vi "KE6221 -- Set Arm Layer Trig Layer Wave Trig Params.vi"(0 "Resource In":refnum<visa-resource-name>, 1 "Check For SCPI Errors? (T)":bool=TRUE, 7 "6221 Arm Trig Wave Trig Params In":T1={"Arm Layer Input Trig Bypassed?"=FALSE, "Arm Layer Input Trig Source"=enum."Immediate", "Arm Layer Input Trig Link Line"=enum."1", "Arm Layer Input Trig Timer Interval (s)"=0.001, "Arm Layer Output Trig Mode"=enum."No Trig Out", "Arm Layer Output Trig Link Line"=enum."1", "Trig Layer Input Trig Source"=enum."Immediate", "Trig Layer Input Trig Link Line"=enum."1", "Trig Layer Output Trig Mode"=enum."No Trig Out", "Trig Layer Output Trig Link Line"=enum."1", "6221 Wave Input Trig Enabled?"=FALSE, "6221 Wave Input Trig Link Line"=enum."None", "6221 Wave Inactive Level (%)"=0.0, "6221 Wave Ingore Input Retrigs?"=FALSE, "6221 Phase Marker Output Trig Enabled?"=FALSE, "6221 Phase Marker (deg)"=180.0, "6221 Phase Marker Output Trig Link Line"=enum."6"} {"6221 Phase Marker (deg)" min=0.0 max=360.0 format="%.3f"; "6221 Wave Inactive Level (%)" min=-100.0 max=100.0 format="%.3p"; "Arm Layer Input Trig Timer Interval (s)" min=0.001 max=99999.999 step=0.001 format="%.3f"}, 11 "error in (no error)":errorcluster) -> (4 "Resource Out (dupl)":refnum<visa-resource-name>, 8 "6221 Arm Trig Wave Trig Params Out":T1={"Arm Layer Input Trig Bypassed?"=FALSE, "Arm Layer Input Trig Source"=enum."Immediate", "Arm Layer Input Trig Link Line"=enum."1", "Arm Layer Input Trig Timer Interval (s)"=0.001, "Arm Layer Output Trig Mode"=enum."No Trig Out", "Arm Layer Output Trig Link Line"=enum."1", "Trig Layer Input Trig Source"=enum."Immediate", "Trig Layer Input Trig Link Line"=enum."1", "Trig Layer Output Trig Mode"=enum."No Trig Out", "Trig Layer Output Trig Link Line"=enum."1", "6221 Wave Input Trig Enabled?"=FALSE, "6221 Wave Input Trig Link Line"=enum."None", "6221 Wave Inactive Level (%)"=0.0, "6221 Wave Ingore Input Retrigs?"=FALSE, "6221 Phase Marker Output Trig Enabled?"=FALSE, "6221 Phase Marker (deg)"=180.0, "6221 Phase Marker Output Trig Link Line"=enum."6"} {"6221 Phase Marker (deg)" min=0.0 max=360.0 format="%.3f"; "6221 Wave Inactive Level (%)" min=-100.0 max=100.0 format="%.3p"; "Arm Layer Input Trig Timer Interval (s)" min=0.001 max=99999.999 step=0.001 format="%.3f"}, 15 "error out":errorcluster)   [LabVIEW 2018, in "Keithley 622x.lvlib"]
doc: "Sets the parameters for the 'Arm' and 'Trigger' layers of the trigger model, and also the trigger parameters for waveform playback. Note that this VI can only be used with the 6221, since the 6220 doesn't support waveform playback."
uses:
  Keithley 622x.lvlib
  Low Level/Typedefs/KE622x -- Trig Source.ctl
  Low Level/Typedefs/KE622x -- Trig Link Line.ctl
  Low Level/Typedefs/KE622x -- Trig Output Mode.ctl
  Low Level/Typedefs/KE622x -- Arm Source.ctl
  Low Level/Typedefs/KE622x -- Arm Output Mode.ctl
  Low Level/Typedefs/KE622x -- Arm Timer Interval.ctl
  6221 Wave/Low Level/Typedefs/KE6221 -- Wave Extern Trig Link In Line.ctl
  6221 Wave/Low Level/Typedefs/KE6221 -- Wave Inactive Level.ctl
  6221 Wave/Low Level/Typedefs/KE6221 -- Wave Phase Marker.ctl
  Typedefs/KE6221 -- Arm Trig Wave Trig Params.ctl
panel:
  out "Num Errors":u32
  out "Errors":string[](array[string])
  # "Arm Layer"
  # "Trig Layer"
  # "KE6221 Wave"
  # "Arm Layer"
  # "Trig Layer"
  # "KE6221 Wave"
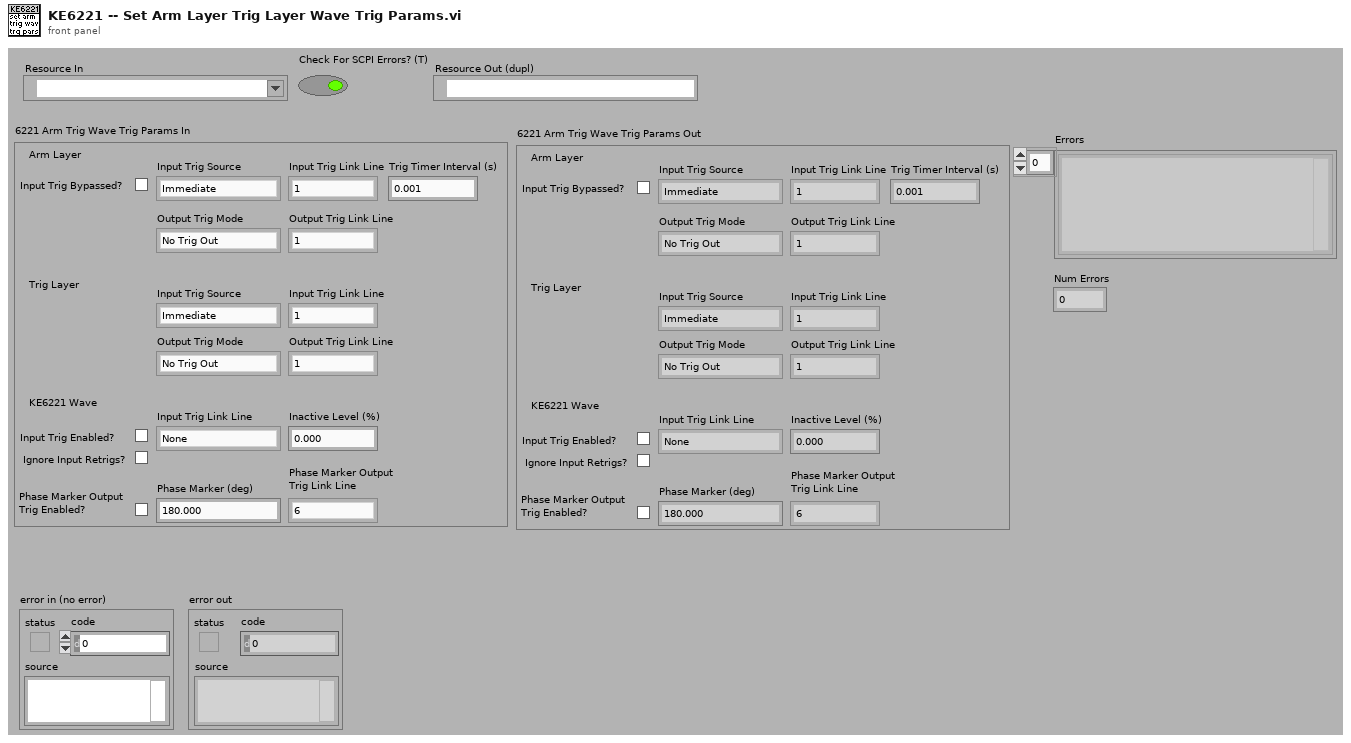
[diagram p1: front panel]
types:
  T1 = typedef "Keithley 622x.lvlib/KE6221 -- Arm Trig Wave Trig Params.ctl" = cluster{"Arm Layer Input Trig Bypassed?":bool, "Arm Layer Input Trig Source":T2, "Arm Layer Input Trig Link Line":T3, "Arm Layer Input Trig Timer Interval (s)":T4, "Arm Layer Output Trig Mode":T5, "Arm Layer Output Trig Link Line":T3, "Trig Layer Input Trig Source":T6, "Trig Layer Input Trig Link Line":T3, "Trig Layer Output Trig Mode":T7, "Trig Layer Output Trig Link Line":T3, "6221 Wave Input Trig Enabled?":bool, "6221 Wave Input Trig Link Line":T8, "6221 Wave Inactive Level (%)":T9, "6221 Wave Ingore Input Retrigs?":bool, "6221 Phase Marker Output Trig Enabled?":bool, "6221 Phase Marker (deg)":T10, "6221 Phase Marker Output Trig Link Line":T3}
  T2 = typedef "Keithley 622x.lvlib/KE622x -- Arm Source.ctl" = enum16{"Immediate", "Bus (*TRG)", "Timer", "Manual", "Trigger Link", "SOT Falling Edge", "SOT Rising Edge", "SOT Either Edge"}
  T3 = typedef "Keithley 622x.lvlib/KE622x -- Trig Link Line.ctl" = enum16{"1", "2", "3", "4", "5", "6"}
  T4 = typedef "Keithley 622x.lvlib/KE622x -- Arm Timer Interval.ctl" = dbl
  T5 = typedef "Keithley 622x.lvlib/KE622x -- Arm Output Mode.ctl" = enum16{"No Trig Out", "Trig Out On Enter Arm", "Trig Out On Exit Arm"}
  T6 = typedef "Keithley 622x.lvlib/KE622x -- Trig Source.ctl" = enum16{"Immediate", "Trigger Link"}
  T7 = typedef "Keithley 622x.lvlib/KE622x -- Trig Output Mode.ctl" = enum16{"No Trig Out", "Source Turn On", "After Source Delay"}
  T8 = typedef "Keithley 622x.lvlib/KE6221 -- Wave Extern Trig Link In Line.ctl" = enum16{"None", "1", "2", "3", "4", "5", "6"}
  T9 = typedef "Keithley 622x.lvlib/KE6221 -- Wave Inactive Level.ctl" = dbl
  T10 = typedef "Keithley 622x.lvlib/KE6221 -- Wave Phase Marker.ctl" = dbl
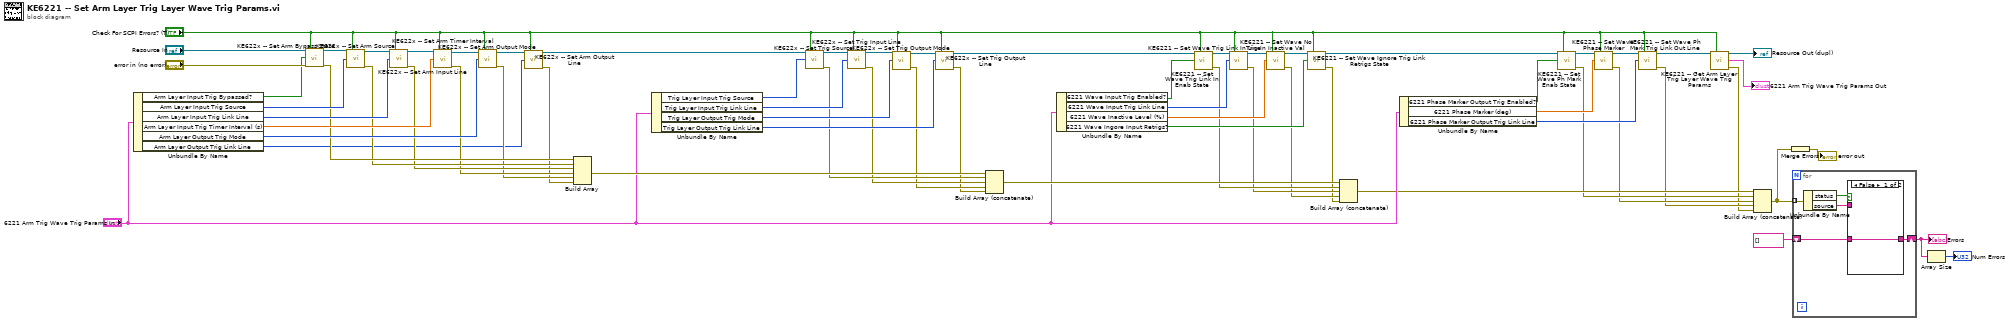
[diagram p0: block diagram]
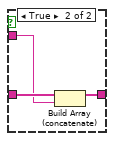
[diagram p2: hidden frame]
diagram:
  n1 = Unbundle By Name("6221 Arm Trig Wave Trig Params In") -> ("Arm Layer Input Trig Bypassed?"=w64:bool, "Arm Layer Input Trig Source"=w62:T2, "Arm Layer Input Trig Link Line"=w60:T3, "Arm Layer Input Trig Timer Interval (s)"=w59:T4, "Arm Layer Output Trig Mode"=w57:T5, "Arm Layer Output Trig Link Line"=w48:T3)
  n2 = call "KE622x -- Set Arm Bypass State.vi"("Resource In"="Resource In", "Check For SCPI Errors? (T)"="Check For SCPI Errors? (T)", "Bypass Arm Layer?"=w64, "error in (no error)"="error in (no error)") -> ("Resource Out (dupl)"=w61:refnum<visa-resource-name>, "error out"=w54:errorcluster)  [unwired: 10 in]
  n3 = call "KE622x -- Set Arm Source.vi"("Resource In"=w61, "Check For SCPI Errors? (T)"="Check For SCPI Errors? (T)", "Arm Source"=w62) -> ("Resource Out (dupl)"=w63:refnum<visa-resource-name>, "error out"=w53:errorcluster)  [unwired: 11 in]
  n4 = call "KE622x -- Set Arm Input Line.vi"("Resource In"=w63, "Check For SCPI Errors? (T)"="Check For SCPI Errors? (T)", "Arm Input Line"=w60) -> ("Resource Out (dupl)"=w58:refnum<visa-resource-name>, "error out"=w52:errorcluster)  [unwired: 11 in]
  n5 = call "KE622x -- Set Arm Timer Interval.vi"("Resource In"=w58, "Check For SCPI Errors? (T)"="Check For SCPI Errors? (T)", "Arm Timer Interval (s)"=w59) -> ("Resource Out (dupl)"=w56:refnum<visa-resource-name>, "error out"=w51:errorcluster)  [unwired: 10 in, 1 out]
  n6 = call "KE622x -- Set Arm Output Mode.vi"("Resource In"=w56, "Check For SCPI Errors? (T)"="Check For SCPI Errors? (T)", "Arm Output Mode"=w57) -> ("Resource Out (dupl)"=w55:refnum<visa-resource-name>, "error out"=w50:errorcluster)  [unwired: 11 in]
  n7 = call "KE622x -- Set Arm Output Line.vi"("Resource In"=w55, "Check For SCPI Errors? (T)"="Check For SCPI Errors? (T)", "Arm Output Line"=w48) -> ("Resource Out (dupl)"=w47:refnum<visa-resource-name>, "error out"=w49:errorcluster)  [unwired: 11 in]
  n8 = Build Array(w54, w53, w52, w51, w50, w49) -> (w39:errorcluster[])
  n9 = Unbundle By Name("6221 Arm Trig Wave Trig Params In") -> ("Trig Layer Input Trig Source"=w46:T6, "Trig Layer Input Trig Link Line"=w44:T3, "Trig Layer Output Trig Mode"=w42:T7, "Trig Layer Output Trig Link Line"=w41:T3)
  n10 = call "KE622x -- Set Trig Source.vi"("Resource In"=w47, "Check For SCPI Errors? (T)"="Check For SCPI Errors? (T)", "Trig Source"=w46) -> ("Resource Out (dupl)"=w45:refnum<visa-resource-name>, "error out"=w38:errorcluster)  [unwired: 11 in]
  n11 = call "KE622x -- Set Trig Input Line.vi"("Resource In"=w45, "Check For SCPI Errors? (T)"="Check For SCPI Errors? (T)", "Trig Input Line"=w44) -> ("Resource Out (dupl)"=w43:refnum<visa-resource-name>, "error out"=w37:errorcluster)  [unwired: 11 in]
  n12 = call "KE622x -- Set Trig Output Mode.vi"("Resource In"=w43, "Check For SCPI Errors? (T)"="Check For SCPI Errors? (T)", "Trig Output Mode"=w42) -> ("Resource Out (dupl)"=w40:refnum<visa-resource-name>, "error out"=w36:errorcluster)  [unwired: 11 in]
  n13 = call "KE622x -- Set Trig Output Line.vi"("Resource In"=w40, "Check For SCPI Errors? (T)"="Check For SCPI Errors? (T)", "Trig Output Line"=w41) -> ("Resource Out (dupl)"=w34:refnum<visa-resource-name>, "error out"=w35:errorcluster)  [unwired: 11 in]
  n14 = Build Array (concatenate)(w39, w38, w37, w36, w35) -> (w26:errorcluster[])
  n15 = Unbundle By Name("6221 Arm Trig Wave Trig Params In") -> ("6221 Wave Input Trig Enabled?"=w33:bool, "6221 Wave Input Trig Link Line"=w32:T8, "6221 Wave Inactive Level (%)"=w29:T9, "6221 Wave Ingore Input Retrigs?"=w28:bool)
  n16 = call "KE6221 -- Set Wave Trig Link In Enab State.vi"("Resource In"=w34, "Check For SCPI Errors? (T)"="Check For SCPI Errors? (T)", "Trig Link In Enabled?"=w33) -> ("Resource Out (dupl)"=w31:refnum<visa-resource-name>, "error out"=w25:errorcluster)  [unwired: 11 in]
  n17 = call "KE6221 -- Set Wave Trig Link In Line.vi"("Resource In"=w31, "Check For SCPI Errors? (T)"="Check For SCPI Errors? (T)", "Trig Link In Line"=w32) -> ("Resource Out (dupl)"=w30:refnum<visa-resource-name>, "error out"=w24:errorcluster)  [unwired: 11 in]
  n18 = call "KE6221 -- Set Wave No Trig In Inactive Val.vi"("Resource In"=w30, "Check For SCPI Errors? (T)"="Check For SCPI Errors? (T)", "Inactive Level In (%)"=w29) -> ("Resource Out (dupl)"=w27:refnum<visa-resource-name>, "error out"=w23:errorcluster)  [unwired: 10 in, 1 out]
  n19 = call "KE6221 -- Set Wave Ignore Trig Link Retrigs State.vi"("Resource In"=w27, "Check For SCPI Errors? (T)"="Check For SCPI Errors? (T)", "Ignore Retrigs?"=w28) -> ("Resource Out (dupl)"=w20:refnum<visa-resource-name>, "error out"=w22:errorcluster)  [unwired: 11 in]
  n20 = Build Array (concatenate)(w26, w25, w24, w23, w22) -> (w14:errorcluster[])
  n21 = Unbundle By Name("6221 Arm Trig Wave Trig Params In") -> ("6221 Phase Marker Output Trig Enabled?"=w19:bool, "6221 Phase Marker (deg)"=w17:T10, "6221 Phase Marker Output Trig Link Line"=w16:T3)
  n22 = call "KE6221 -- Set Wave Ph Mark Enab State.vi"("Resource In"=w20, "Check For SCPI Errors? (T)"="Check For SCPI Errors? (T)", "Phase Marker Enabled?"=w19) -> ("Resource Out (dupl)"=w18:refnum<visa-resource-name>, "error out"=w13:errorcluster)  [unwired: 11 in]
  n23 = call "KE6221 -- Set Wave Phase Marker.vi"("Resource In"=w18, "Check For SCPI Errors? (T)"="Check For SCPI Errors? (T)", "Phase Marker In (deg)"=w17) -> ("Resource Out (dupl)"=w15:refnum<visa-resource-name>, "error out"=w12:errorcluster)  [unwired: 10 in, 1 out]
  n24 = call "KE6221 -- Set Wave Ph Mark Trig Link Out Line.vi"("Resource In"=w15, "Check For SCPI Errors? (T)"="Check For SCPI Errors? (T)", "Trig Link Out Line"=w16) -> ("Resource Out (dupl)"=w10:refnum<visa-resource-name>, "error out"=w11:errorcluster)  [unwired: 11 in]
  n25 = call "KE6221 -- Get Arm Layer Trig Layer Wave Trig Params.vi"("Resource In"=w10, "Check For SCPI Errors? (T)"="Check For SCPI Errors? (T)") -> ("Resource Out (dupl)"=→"Resource Out (dupl)":refnum<visa-resource-name>, "6221 Arm Trig Wave Trig Params"=→"6221 Arm Trig Wave Trig Params Out":T1, "error out"=w8:errorcluster)  [unwired: 11 in]
  n26 = Build Array (concatenate)(w14, w13, w12, w11, w8) -> (w4:errorcluster[])
  n27 = Merge Errors(w4) -> (→"error out":errorcluster)
  n28 = for {
    tunnel: w4 -> [w71] mode=indexing
    shift-right: [w67] -> w1
    shift-left: string[] [] -> [w68]
    n29 = Unbundle By Name(w71) -> ("status"=w70:bool, "source"=w69:string)
    n30 = case shown="False" w70 {
      tunnel: w69 -> [_ w74]
      tunnel: w68 -> [w72 w75]
      tunnel: [w72 w73] -> w67
      frame False {
      }
      frame True {
        n31 = Build Array (concatenate)(w75, w74) -> (w73:string[])
      }
    }
  }
  "Errors" <- w1
  n32 = Array Size(array=w1) -> (size(s)=→"Num Errors":i32)
